vi "ComputeFlowrates.vi"(4 "minFlowrate (l/min)":dbl min=0.0 max=360.0 step=1.0 format="%.2f", 5 "Pressure channel":string, 6 "maxFlowrate (l/min)":dbl min=0.0 max=360.0 step=1.0 format="%.2f", 7 "Temperature channel":string, 9 "C_dem:(%)":dbl, 10 "Q_dem[Total]:(l/min)":dbl, 11 "DataBus in":T1 {"RhoTrace" format="%.3gg/l"; "RhoCarrier" format="%.3gg/l"; "InactiveC2H6MFCs"."mDot" format="%_4g"; "InactiveC2H6MFCs"."Setpoint" format="%.2g"; "InactiveC2H6MFCs"."MFCcapability"."MaxMdot" format="%_4g"; "InactiveC2H6MFCs"."MFCcapability"."MinMdot" format="%_4g"; "ActiveC2H6MFCs"."mDot" format="%_4g"; "ActiveC2H6MFCs"."Setpoint" format="%.2g"; "ActiveC2H6MFCs"."MFCcapability"."MaxMdot" format="%_4g"; "ActiveC2H6MFCs"."MFCcapability"."MinMdot" format="%_4g"; "InactiveN2MFCs"."mDot" format="%_4g"; "InactiveN2MFCs"."Setpoint" format="%.2g"; "InactiveN2MFCs"."MFCcapability"."MaxMdot" format="%_4g"; "InactiveN2MFCs"."MFCcapability"."MinMdot" format="%_4g"; "ActiveN2MFCs"."mDot" format="%_4g"; "ActiveN2MFCs"."Setpoint" format="%.2g"; "ActiveN2MFCs"."MFCcapability"."MaxMdot" format="%_4g"; "ActiveN2MFCs"."MFCcapability"."MinMdot" format="%_4g"; "C2H6MFCs"."mDot" format="%_4g"; "C2H6MFCs"."Setpoint" format="%.2g"; "C2H6MFCs"."MFCcapability"."MaxMdot" format="%_4g"; "C2H6MFCs"."MFCcapability"."MinMdot" format="%_4g"; "N2MFCs"."mDot" format="%_4g"; "N2MFCs"."Setpoint" format="%.2g"; "N2MFCs"."MFCcapability"."MaxMdot" format="%_4g"; "N2MFCs"."MFCcapability"."MinMdot" format="%_4g"; "QdemCarrier" format="%.2pl/min"; "QdemTrace" format="%.2pl/min"; "MdotCarrier" format="%_4pg/min"; "MdotTrace" format="%_4pg/min"; "releaseTemp" format="%#_gC"; "releasePress" format="%#_gmBar"}) -> (1 "errorString":string, 3 "DataBus out":T1 {"RhoTrace" format="%.3gg/l"; "RhoCarrier" format="%.3gg/l"; "InactiveC2H6MFCs"."mDot" format="%_4g"; "InactiveC2H6MFCs"."Setpoint" format="%.2g"; "InactiveC2H6MFCs"."MFCcapability"."MaxMdot" format="%_4g"; "InactiveC2H6MFCs"."MFCcapability"."MinMdot" format="%_4g"; "ActiveC2H6MFCs"."mDot" format="%_4g"; "ActiveC2H6MFCs"."Setpoint" format="%.2g"; "ActiveC2H6MFCs"."MFCcapability"."MaxMdot" format="%_4g"; "ActiveC2H6MFCs"."MFCcapability"."MinMdot" format="%_4g"; "InactiveN2MFCs"."mDot" format="%_4g"; "InactiveN2MFCs"."Setpoint" format="%.2g"; "InactiveN2MFCs"."MFCcapability"."MaxMdot" format="%_4g"; "InactiveN2MFCs"."MFCcapability"."MinMdot" format="%_4g"; "ActiveN2MFCs"."mDot" format="%_4g"; "ActiveN2MFCs"."Setpoint" format="%.2g"; "ActiveN2MFCs"."MFCcapability"."MaxMdot" format="%_4g"; "ActiveN2MFCs"."MFCcapability"."MinMdot" format="%_4g"; "C2H6MFCs"."mDot" format="%_4g"; "C2H6MFCs"."Setpoint" format="%.2g"; "C2H6MFCs"."MFCcapability"."MaxMdot" format="%_4g"; "C2H6MFCs"."MFCcapability"."MinMdot" format="%_4g"; "N2MFCs"."mDot" format="%_4g"; "N2MFCs"."Setpoint" format="%.2g"; "N2MFCs"."MFCcapability"."MaxMdot" format="%_4g"; "N2MFCs"."MFCcapability"."MinMdot" format="%_4g"; "QdemCarrier" format="%.2pl/min"; "QdemTrace" format="%.2pl/min"; "MdotCarrier" format="%_4pg/min"; "MdotTrace" format="%_4pg/min"; "releaseTemp" format="%#_gC"; "releasePress" format="%#_gmBar"})   [LabVIEW 2021]
uses:
  AalborgServerData.ctl
  MFCdescription.ctl
  MFCcapability.ctl
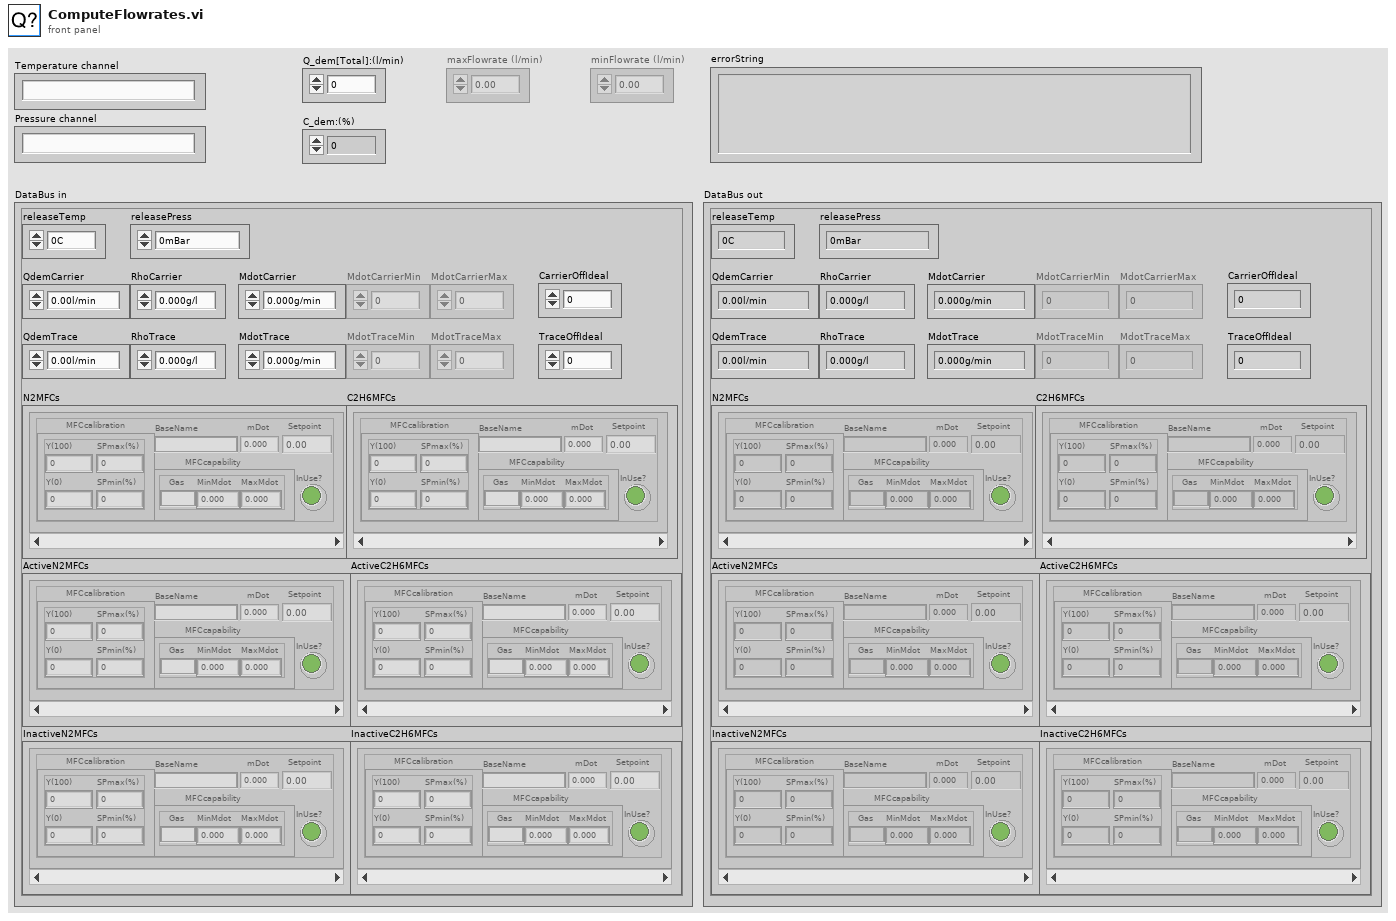
[diagram p1: front panel]
types:
  T1 = typedef "AalborgServerData.ctl" = cluster{"releaseTemp":dbl, "releasePress":dbl, "QdemCarrier":dbl, "QdemTrace":dbl, "MdotCarrier":dbl, "MdotCarrierMin":dbl, "MdotCarrierMax":dbl, "MdotTrace":dbl, "MdotTraceMin":dbl, "MdotTraceMax":dbl, "N2MFCs":T2[], "C2H6MFCs":T2[], "CarrierOffIdeal":dbl, "TraceOffIdeal":dbl, "ActiveN2MFCs":T2[], "InactiveN2MFCs":T2[], "ActiveC2H6MFCs":T2[], "InactiveC2H6MFCs":T2[], "RhoCarrier":dbl, "RhoTrace":dbl}
  T2 = typedef "MFCdescription.ctl" = cluster{"BaseName":string, "MFCcalibration":cluster{"Y(100)":dbl, "Y(0)":dbl, "SPmin(%)":dbl, "SPmax(%)":dbl}, "MFCcapability":T3, "InUse?":bool, "Setpoint":dbl, "mDot":dbl}
  T3 = typedef "MFCcapability.ctl" = cluster{"Gas":string, "MinMdot":dbl, "MaxMdot":dbl}
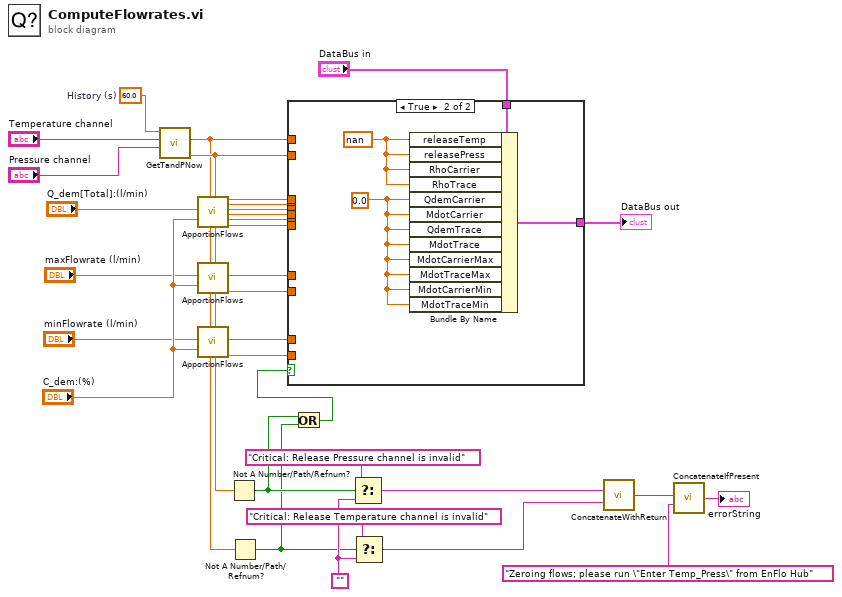
[diagram p0: block diagram]
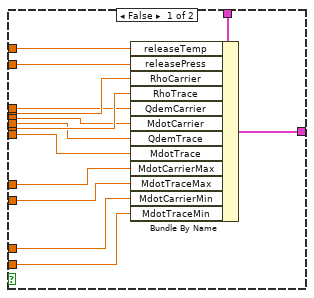
[diagram p2: hidden frame]
diagram:
  w11 = ""
  w28 = 60.0  # History (s)
  n1 = call "GetTandPNow.vi"("Pressure channel"="Pressure channel", "Temperature channel"="Temperature channel", "History (s)"=w28) -> ("Press (mBar)"=w8:dbl, "Temp (C)"=w7:dbl)  [unwired: 7 in]
  n2 = call "ApportionFlows.vi"("Q[Total]:(l/min)"="Q_dem[Total]:(l/min)", "C:(%)"="C_dem:(%)", "Temp (C)"=w7, "Press (mBar)"=w8) -> ("Q[N2]:(l/min)"=w21:dbl, "Rho[N2]:(kg/l)"=w23:dbl, "Mdot[N2]:(g/min)"=w20:dbl, "Q[Ethane]:(l/min)"=w19:dbl, "Rho[Ethane]:(kg/l)"=w22:dbl, "Mdot[Ethane]:(g/min)"=w18:dbl)  [unwired: 10 in]
  n3 = call "ApportionFlows.vi"("Q[Total]:(l/min)"="maxFlowrate (l/min)", "C:(%)"="C_dem:(%)", "Temp (C)"=w7, "Press (mBar)"=w8) -> ("Mdot[N2]:(g/min)"=w17:dbl, "Mdot[Ethane]:(g/min)"=w16:dbl)  [unwired: 10 in, 4 out]
  n4 = call "ApportionFlows.vi"("Q[Total]:(l/min)"="minFlowrate (l/min)", "C:(%)"="C_dem:(%)", "Temp (C)"=w7, "Press (mBar)"=w8) -> ("Mdot[N2]:(g/min)"=w15:dbl, "Mdot[Ethane]:(g/min)"=w14:dbl)  [unwired: 10 in, 4 out]
  n5 = Not A Number/Path/Refnum?(number/path/refnum=w8) -> (NaN/Path/Refnum?=w6:bool)
  n6 = Not A Number/Path/Refnum?(number/path/refnum=w7) -> (NaN/Path/Refnum?=w5:bool)
  n7 = Or(x=w6, y=w5) -> (x .or. y?=w4:bool)
  n8 = case shown="True" w4 {
    tunnel: [w46 w50] -> w30
    tunnel: "DataBus in" -> [w45 w49]
    tunnel: w23 -> [w44 _]
    tunnel: w22 -> [w43 _]
    tunnel: w21 -> [w42 _]
    tunnel: w20 -> [w41 _]
    tunnel: w19 -> [w40 _]
    tunnel: w18 -> [w39 _]
    tunnel: w17 -> [w38 _]
    tunnel: w16 -> [w37 _]
    tunnel: w15 -> [w36 _]
    tunnel: w14 -> [w35 _]
    tunnel: w8 -> [w34 _]
    tunnel: w7 -> [w33 _]
    frame False {
      n9 = Bundle By Name(cluster=w45, "releaseTemp"=w33, "releasePress"=w34, "RhoCarrier"=w44, "RhoTrace"=w43, "QdemCarrier"=w42, "MdotCarrier"=w41, "QdemTrace"=w40, "MdotTrace"=w39, "MdotCarrierMax"=w38, "MdotTraceMax"=w37, "MdotCarrierMin"=w36, "MdotTraceMin"=w35) -> (w46:T1)
    }
    frame True {
      w47 = 0.0
      w48 = nan
      n10 = Bundle By Name(cluster=w49, "releaseTemp"=w48, "releasePress"=w48, "RhoCarrier"=w48, "RhoTrace"=w48, "QdemCarrier"=w47, "MdotCarrier"=w47, "QdemTrace"=w47, "MdotTrace"=w47, "MdotCarrierMax"=w47, "MdotTraceMax"=w47, "MdotCarrierMin"=w47, "MdotTraceMin"=w47) -> (w50:T1)
    }
  }
  "DataBus out" <- w30
  n11 = Select(t="Critical: Release Pressure channel is invalid", s=w6, f=w11) -> (s? t:f=w10:string)
  n12 = Select(t="Critical: Release Temperature channel is invalid", s=w5, f=w11) -> (s? t:f=w9:string)
  n13 = call "ConcatenateWithReturn.vi"("baseString"=w10, "additionalString"=w9) -> ("outputString"=w3:string)  [unwired: 13 in]
  n14 = call "ConcatenateIfPresent.vi"("prependString"=w3, "appendString"="Zeroing flows; please run \"Enter Temp_Press\" from EnFlo Hub") -> ("outputString"=→"errorString":string)  [unwired: 13 in]
